vi "SCLN_ExampleClient.vi"() -> ()   [LabVIEW 2015]
panel:
  out "Mean2":dbl format="%#.1g"
  out "Mean1":dbl format="%#.1g"
  out "Command sent 2":string
  out "Command sent 1":string
  out "Compare 2":bool
  out "Compare 1":bool
  out "CLT2":errorcluster={"status"=TRUE, "code"=7, "source"="File/Directory Info in Open Config Data.vi->SCLN_ReadConfig.vi->SCLN_InitClient.vi->SCLN_ExampleClient.vi"}
  out "CLT1":errorcluster={"status"=TRUE, "code"=7, "source"="File/Directory Info in Open Config Data.vi->SCLN_ReadConfig.vi->SCLN_InitClient.vi->SCLN_ExampleClient.vi"}
  out "Connected 2":bool
  out "Connected 1":bool
  out "Max 2":i32
  out "Max 1":i32
  out "Loop 2":i32(graph)
  out "Loop 1":i32(graph)
  in  "stop":bool
  out "Error 2":errorcluster
  out "Error 1":errorcluster
  out "Response 2":string
  in  "Command 2":string="wnbadj 38462395 qli2u34u c12837vb asdfjh "
  out "Response 1":string
  in  "Command 1":string="sjdgha kjs sj sdifjsklif alkda  oaidpaqoidkp "
  in  "Config Filename":path=path "C:/scln_oe/SCLN/config/examples.cfg"
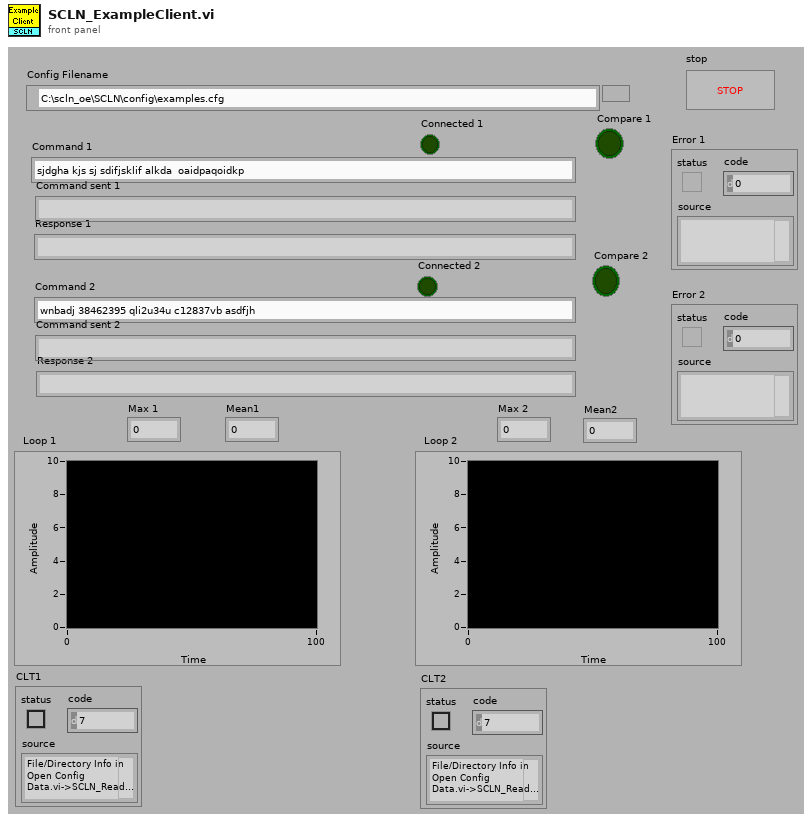
[diagram p1: front panel]
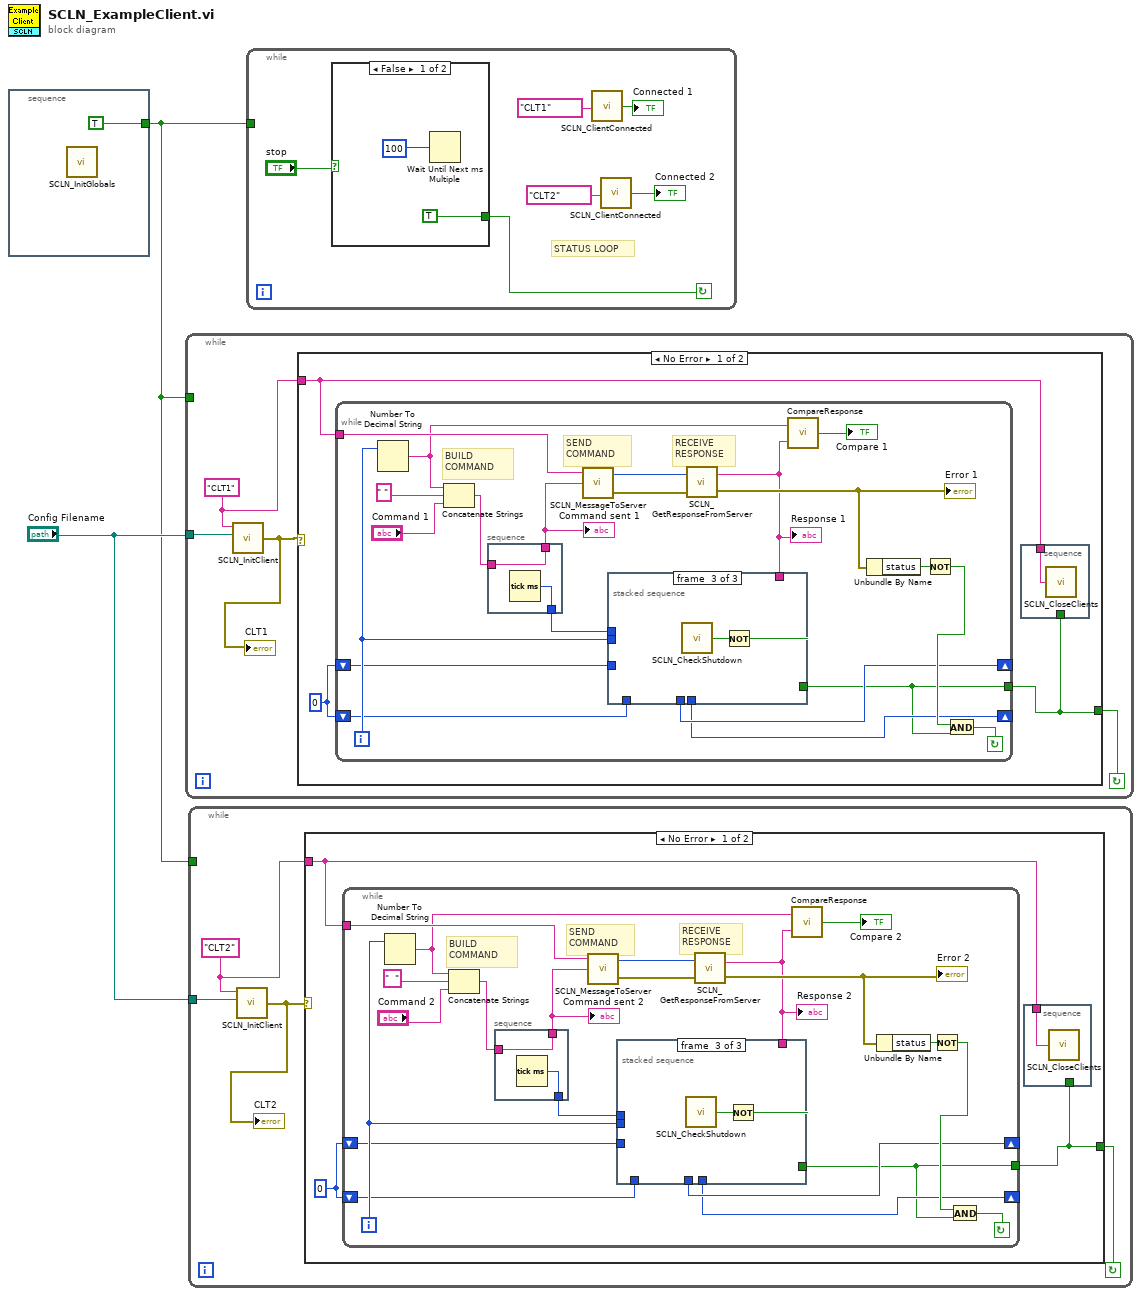
[diagram p0: block diagram]
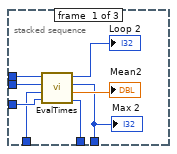
[diagram p2: hidden frame]
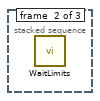
[diagram p3: hidden frame]
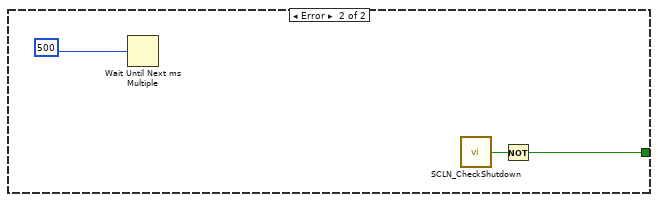
[diagram p4: hidden frame]
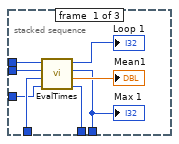
[diagram p5: hidden frame]
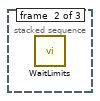
[diagram p6: hidden frame]
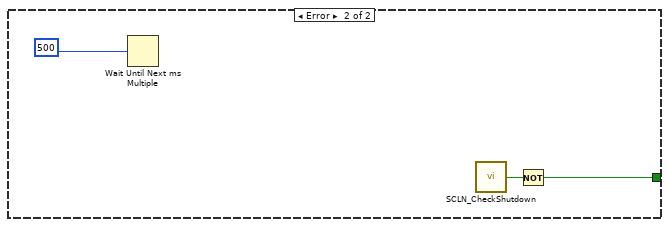
[diagram p7: hidden frame]
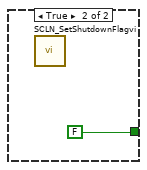
[diagram p8: hidden frame]
diagram:
  n1 = stacked-sequence {
    tunnel: [TRUE] -> w1
    frame #0 {
      n2 = call "SCLN_InitGlobals.vi"() -> ()  [unwired: 1 in]
    }
  }
  n3 = while {
    tunnel: "Config Filename" -> [w7]
    tunnel: w1 -> [_]
    stop <- w6 continue-if-true
    w4 = "CLT1"
    n4 = call "SCLN_InitClient.vi"("Config File Name"=w7, "Server Name"=w4) -> ("error out"=w5:errorcluster)  [unwired: 2 in]
    "CLT1" <- w5
    n5 = case shown="No Error" w5 {
      tunnel: [w10 w45] -> w6
      tunnel: w4 -> [w9 _]
      frame No Error {
        w8 = 0
        n6 = while {
          shift-right: [w14] -> _
          shift-left: w8 -> [w18]
          tunnel: [w13] -> w10
          tunnel: w9 -> [w25]
          shift-right: [w16] -> _
          shift-left: w8 -> [w17]
          i -> [w19]
          stop <- w26 continue-if-true
          # "BUILD\nCOMMAND"
          # "RECEIVE\nRESPONSE"
          # "SEND\nCOMMAND"
          n7 = Number To Decimal String(number=w19) -> (decimal integer string=w24:string)  [unwired: 1 in]
          n8 = Concatenate Strings(w24, " ", "Command 1") -> (w31:string)
          n9 = stacked-sequence {
            tunnel: w31 -> [w44]
            tunnel: [w44] -> w23
            tunnel: [w43] -> w20
            frame #0 {
              n10 = Tick Count (ms)() -> (millisecond timer value=w43:u32)
            }
          }
          "Command sent 1" <- w23
          n11 = call "SCLN_MessageToServer.vi"("Message"=w23, "Server Name"=w25) -> ("error out"=w29:errorcluster, "Index for Response"=w30:i32)  [unwired: 1 in]
          n12 = call "SCLN_GetResponseFromServer.vi"("error in (no error)"=w29, "Index for Response"=w30) -> ("error out"=w15:errorcluster, "Message"=w12:string)
          "Error 1" <- w15
          "Response 1" <- w12
          n13 = stacked-sequence {
            tunnel: w12 -> [_ _ _]
            tunnel: w20 -> [w40 _ _]
            tunnel: w19 -> [w39 _ _]
            tunnel: w18 -> [w38 _ _]
            tunnel: w17 -> [w37 _ _]
            tunnel: [w36 _ _] -> w16
            tunnel: [w33 _ _] -> w14
            tunnel: [_ _ w41] -> w13
            frame #0 {
              n14 = call "EvalTimes.vi"("Total_Delta_In"=w37, "Max_In"=w38, "Iteration"=w39, "Init_Time"=w40) -> ("Total_Delta_Out"=w36:i32, "Mean"=→"Mean1":dbl, "Max_Out"=w33:i32, "Delta"=→"Loop 1":i32)
              "Max 1" <- w33
            }
            frame #1 {
              n15 = call "WaitLimits.vi"() -> ()  [unwired: 4 in]
            }
            frame #2 {
              n16 = call "SCLN_CheckShutdown.vi"() -> ("Shutdown"=w42:bool)
              n17 = Not(x=w42) -> (.not. x?=w41:bool)
            }
          }
          n18 = call "CompareResponse.vi"("Response"=w12, "Number"=w24) -> ("Not Equal"=→"Compare 1":bool)
          n19 = Unbundle By Name(w15) -> ("status"=w28:bool)
          n20 = Not(x=w28) -> (.not. x?=w27:bool)
          n21 = And(x=w27, y=w13) -> (x .and. y?=w26:bool)
        }
        n22 = stacked-sequence {
          tunnel: w10 -> [_]
          tunnel: w9 -> [w11]
          frame #0 {
            n23 = call "SCLN_CloseClients.vi"("Server Name"=w11) -> ()
          }
        }
      }
      frame Error {
        n24 = Wait Until Next ms Multiple(millisecond multiple=500) -> ()  [unwired: 1 out]
        n25 = call "SCLN_CheckShutdown.vi"() -> ("Shutdown"=w47:bool)
        n26 = Not(x=w47) -> (.not. x?=w45:bool)
      }
    }
  }
  n27 = while {
    tunnel: "Config Filename" -> [w51]
    tunnel: w1 -> [_]
    stop <- w50 continue-if-true
    w49 = "CLT2"
    n28 = call "SCLN_InitClient.vi"("Config File Name"=w51, "Server Name"=w49) -> ("error out"=w48:errorcluster)  [unwired: 2 in]
    "CLT2" <- w48
    n29 = case shown="No Error" w48 {
      tunnel: [w54 w89] -> w50
      tunnel: w49 -> [w53 _]
      frame No Error {
        w52 = 0
        n30 = while {
          shift-right: [w58] -> _
          shift-left: w52 -> [w60]
          tunnel: [w57] -> w54
          tunnel: w53 -> [w67]
          shift-right: [w59] -> _
          shift-left: w52 -> [w61]
          i -> [w62]
          stop <- w68 continue-if-true
          # "BUILD\nCOMMAND"
          # "RECEIVE\nRESPONSE"
          # "SEND\nCOMMAND"
          n31 = Number To Decimal String(number=w62) -> (decimal integer string=w66:string)  [unwired: 1 in]
          n32 = Concatenate Strings(w66, "  ", "Command 2") -> (w75:string)
          n33 = stacked-sequence {
            tunnel: w75 -> [w88]
            tunnel: [w88] -> w65
            tunnel: [w87] -> w63
            frame #0 {
              n34 = Tick Count (ms)() -> (millisecond timer value=w87:u32)
            }
          }
          "Command sent 2" <- w65
          n35 = call "SCLN_MessageToServer.vi"("Message"=w65, "Server Name"=w67) -> ("error out"=w73:errorcluster, "Index for Response"=w74:i32)  [unwired: 1 in]
          n36 = call "SCLN_GetResponseFromServer.vi"("error in (no error)"=w73, "Index for Response"=w74) -> ("error out"=w71:errorcluster, "Message"=w56:string)
          "Error 2" <- w71
          "Response 2" <- w56
          n37 = stacked-sequence {
            tunnel: w56 -> [_ _ _]
            tunnel: w63 -> [w84 _ _]
            tunnel: w62 -> [w83 _ _]
            tunnel: w61 -> [w82 _ _]
            tunnel: w60 -> [w81 _ _]
            tunnel: [w80 _ _] -> w59
            tunnel: [w77 _ _] -> w58
            tunnel: [_ _ w85] -> w57
            frame #0 {
              n38 = call "EvalTimes.vi"("Total_Delta_In"=w82, "Max_In"=w81, "Iteration"=w83, "Init_Time"=w84) -> ("Total_Delta_Out"=w80:i32, "Mean"=→"Mean2":dbl, "Max_Out"=w77:i32, "Delta"=→"Loop 2":i32)
              "Max 2" <- w77
            }
            frame #1 {
              n39 = call "WaitLimits.vi"() -> ()  [unwired: 4 in]
            }
            frame #2 {
              n40 = call "SCLN_CheckShutdown.vi"() -> ("Shutdown"=w86:bool)
              n41 = Not(x=w86) -> (.not. x?=w85:bool)
            }
          }
          n42 = call "CompareResponse.vi"("Response"=w56, "Number"=w66) -> ("Not Equal"=→"Compare 2":bool)
          n43 = Unbundle By Name(w71) -> ("status"=w70:bool)
          n44 = Not(x=w70) -> (.not. x?=w69:bool)
          n45 = And(x=w69, y=w57) -> (x .and. y?=w68:bool)
        }
        n46 = stacked-sequence {
          tunnel: w54 -> [_]
          tunnel: w53 -> [w55]
          frame #0 {
            n47 = call "SCLN_CloseClients.vi"("Server Name"=w55) -> ()
          }
        }
      }
      frame Error {
        n48 = Wait Until Next ms Multiple(millisecond multiple=500) -> ()  [unwired: 1 out]
        n49 = call "SCLN_CheckShutdown.vi"() -> ("Shutdown"=w91:bool)
        n50 = Not(x=w91) -> (.not. x?=w89:bool)
      }
    }
  }
  n51 = while {
    tunnel: w1 -> [_]
    stop <- w92 continue-if-true
    # "STATUS LOOP"
    n52 = case shown="False" "stop" {
      tunnel: [TRUE FALSE] -> w92
      frame False {
        n53 = Wait Until Next ms Multiple(millisecond multiple=100) -> ()  [unwired: 1 out]
      }
      frame True {
        n54 = call "SCLN_SetShutdownFlagvi.vi"() -> ()  [unwired: 1 in]
      }
    }
    n55 = call "SCLN_ClientConnected.vi"("Server Name"="CLT1") -> ("Connected"=→"Connected 1":bool)
    n56 = call "SCLN_ClientConnected.vi"("Server Name"="CLT2") -> ("Connected"=→"Connected 2":bool)
  }
